vi "Viavi - Get Measure Data.vi"(8 "error in (no error)":errorcluster, 9 "Selected Wavelength":bool, 10 "Warning/Error Params":T3={"IL Param"={"Warning High"=inf, "Warning Low"=-inf, "Fail High"=inf, "Fail Low"=-inf, "Display Precision"=0}, "RL Param"={"Warning High"=inf, "Warning Low"=-inf, "Fail High"=inf, "Fail Low"=-inf, "Display Precision"=0}, "RL2 Param"={"Warning High"=inf, "Warning Low"=-inf, "Fail High"=inf, "Fail Low"=-inf, "Display Precision"=0}, "Power Param"={"Warning High"=inf, "Warning Low"=-inf, "Fail High"=inf, "Fail Low"=-inf, "Display Precision"=0}, "Length Param"={"Warning High"=inf, "Warning Low"=-inf, "Fail High"=inf, "Fail Low"=-inf, "Display Precision"=0}}, 11 "Viavi - strictRefs":T1) -> (0 "error out":errorcluster, 1 "Failure Output":string, 3 "Output Cluster":T2)   [LabVIEW 2017]
uses:
  Controls/Viavi - objectRefs.ctl
  <instrlib>/Viavi mORL-A1/Viavi mORL-A1.lvlib
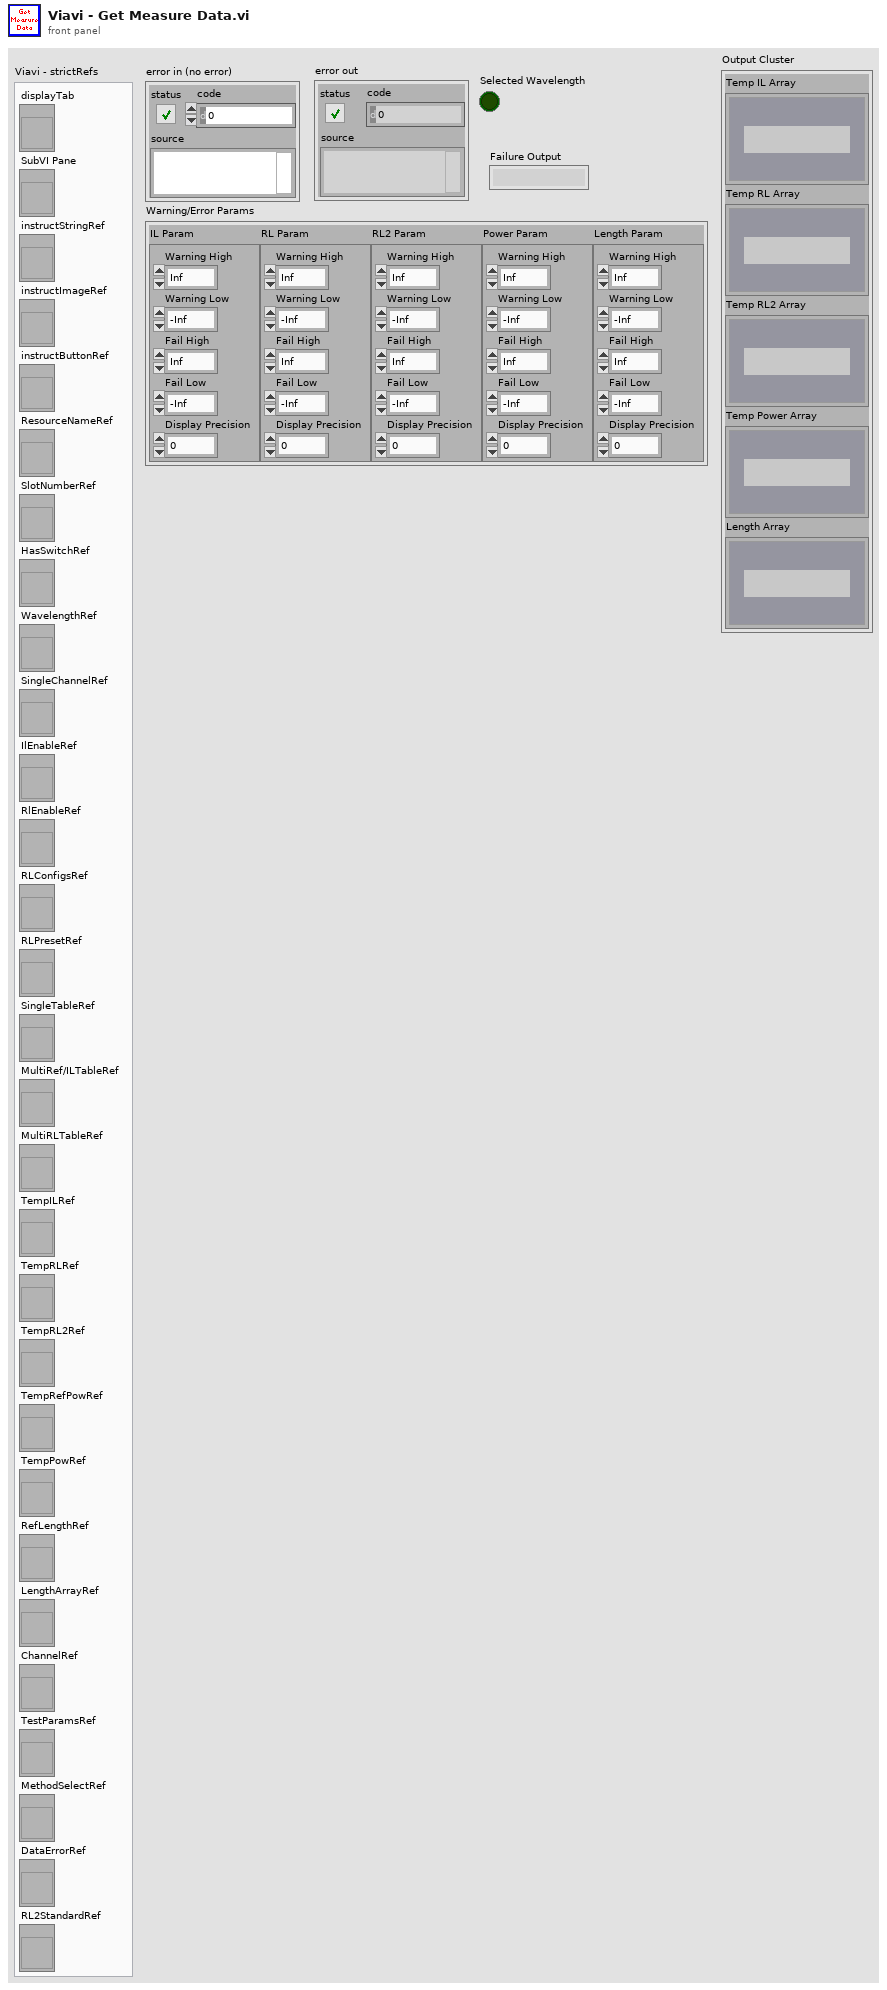
[diagram p1: front panel]
types:
  T1 = typedef "Viavi - objectRefs.ctl" = cluster{"displayTab":refnum<vi>, "SubVI Pane":refnum<vi>, "instructStringRef":refnum<vi>, "instructImageRef":refnum<vi>, "instructButtonRef":refnum<vi>, "ResourceNameRef":refnum<vi>, "SlotNumberRef":refnum<vi>, "HasSwitchRef":refnum<vi>, "WavelengthRef":refnum<vi>, "SingleChannelRef":refnum<vi>, "IlEnableRef":refnum<vi>, "RlEnableRef":refnum<vi>, "RLConfigsRef":refnum<vi>, "RLPresetRef":refnum<vi>, "SingleTableRef":refnum<vi>, "MultiRef/ILTableRef":refnum<vi>, "MultiRLTableRef":refnum<vi>, "TempILRef":refnum<vi>, "TempRLRef":refnum<vi>, "TempRL2Ref":refnum<vi>, "TempRefPowRef":refnum<vi>, "TempPowRef":refnum<vi>, "RefLengthRef":refnum<vi>, "LengthArrayRef":refnum<vi>, "ChannelRef":refnum<vi>, "TestParamsRef":refnum<vi>, "MethodSelectRef":refnum<vi>, "DataErrorRef":refnum<vi>, "RL2StandardRef":refnum<vi>}
  T2 = cluster{"Temp IL Array":cluster{"String":string, "Warning":bool, "Fail":bool, "Numeric":dbl}[], "Temp RL Array":cluster{"String":string, "Warning":bool, "Fail":bool, "Numeric":dbl}[], "Temp RL2 Array":cluster{"String":string, "Warning":bool, "Fail":bool, "Numeric":dbl}[], "Temp Power Array":cluster{"String":string, "Warning":bool, "Fail":bool, "Numeric":dbl}[], "Length Array":cluster{"String":string, "Warning":bool, "Fail":bool, "Numeric":dbl}[]}
  T3 = cluster{"IL Param":cluster{"Warning High":dbl, "Warning Low":dbl, "Fail High":dbl, "Fail Low":dbl, "Display Precision":i32}, "RL Param":cluster{"Warning High":dbl, "Warning Low":dbl, "Fail High":dbl, "Fail Low":dbl, "Display Precision":i32}, "RL2 Param":cluster{"Warning High":dbl, "Warning Low":dbl, "Fail High":dbl, "Fail Low":dbl, "Display Precision":i32}, "Power Param":cluster{"Warning High":dbl, "Warning Low":dbl, "Fail High":dbl, "Fail Low":dbl, "Display Precision":i32}, "Length Param":cluster{"Warning High":dbl, "Warning Low":dbl, "Fail High":dbl, "Fail Low":dbl, "Display Precision":i32}}
  T4 = enum32{"Left Anchor", "Right Anchor", "Center Anchor", "Left/Right Anchor", "Custom"}
  T5 = cluster{"String":string, "Warning":bool, "Fail":bool, "Numeric":dbl}[]
  T6 = cluster{"Measurement Mode":bool, "Enable RL2":bool, "RL1 Anchor Point":enum32{"Left DUT Connection", "Right DUT Connection", "Center on DUT"}, "RL1 Measure Points":cluster{"RL1 Left":dbl, "RL1 Right":dbl}, "RL2 Anchor Point":enum32{"Left DUT Connection", "Right DUT Connection", "Center on DUT"}, "RL2 Measure Points":cluster{"RL2 Left":dbl, "RL2 Right":dbl}}
  T7 = enum32{"Left DUT Connection", "Right DUT Connection", "Center on DUT"}
  T8 = cluster{"String":string, "Warning":bool, "Fail":bool, "Numeric":dbl}
  T9 = enum32{"Left/Right Anchor", "Left Anchor", "Right Anchor", "Center Anchor", "Custom"}
  T10 = cluster{"Warning High":dbl, "Warning Low":dbl, "Fail High":dbl, "Fail Low":dbl, "Display Precision":i32}
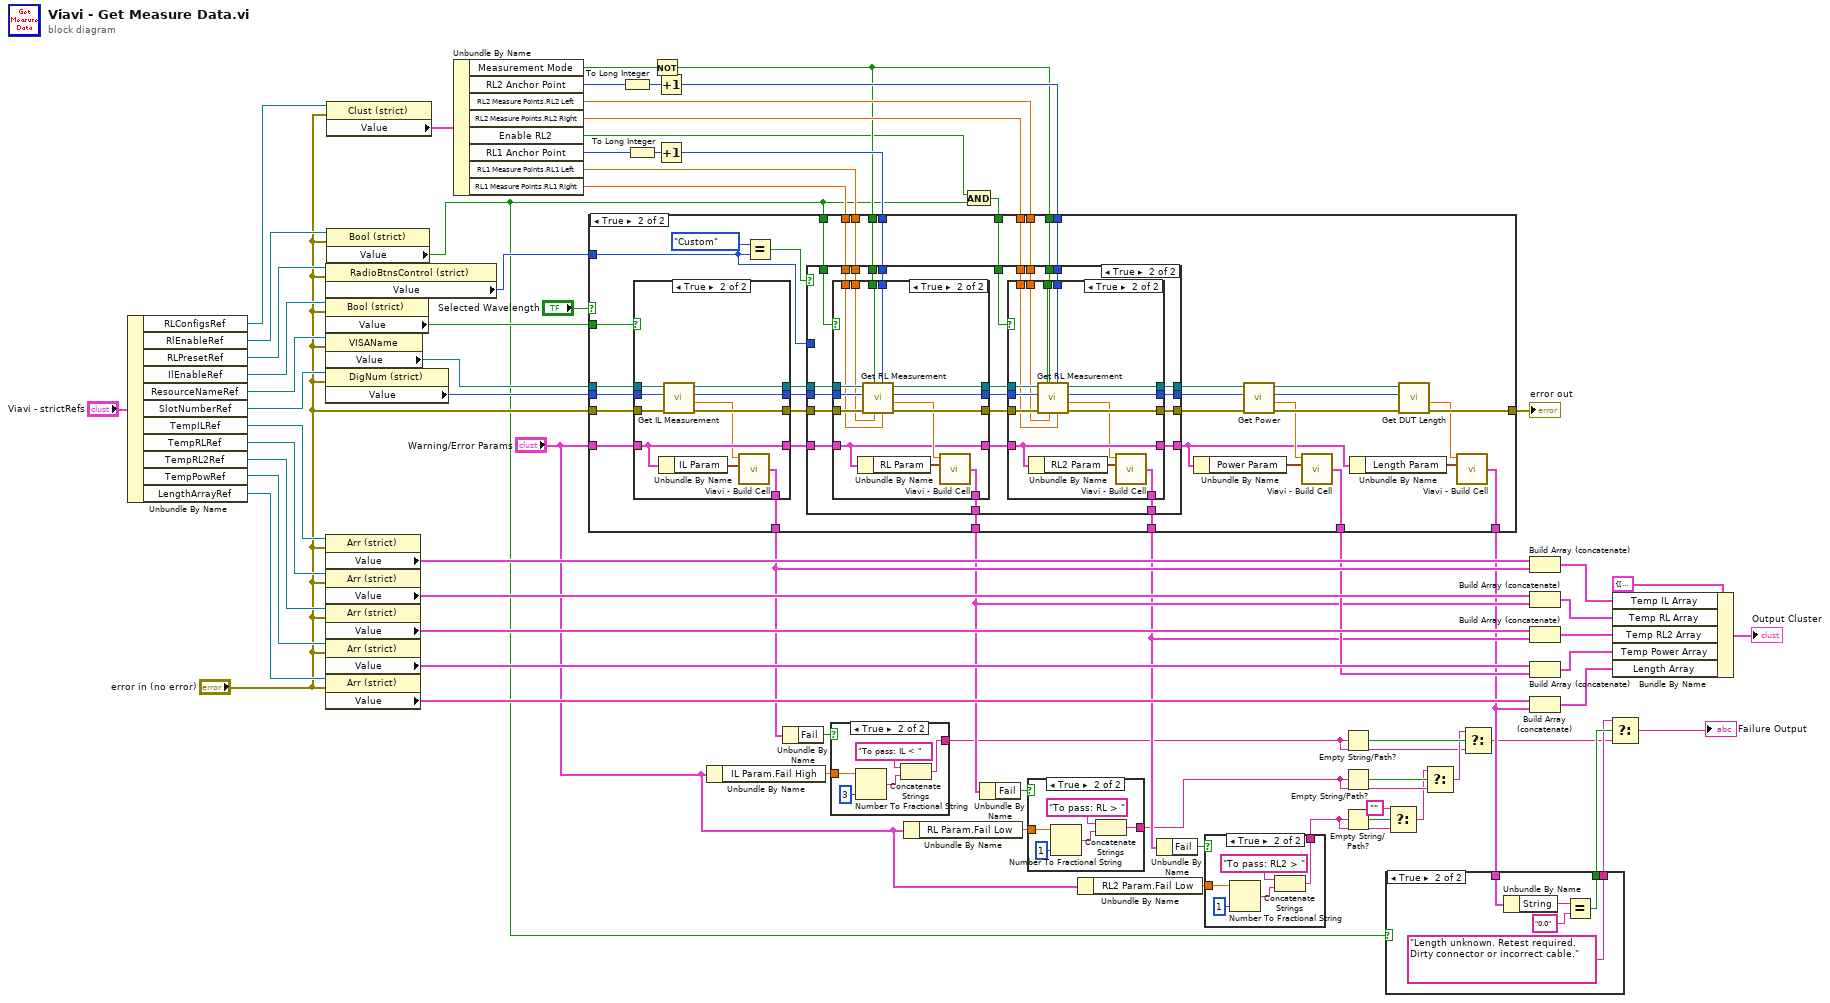
[diagram p0: block diagram]
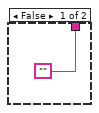
[diagram p3: hidden frame]
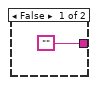
[diagram p4: hidden frame]
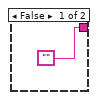
[diagram p5: hidden frame]
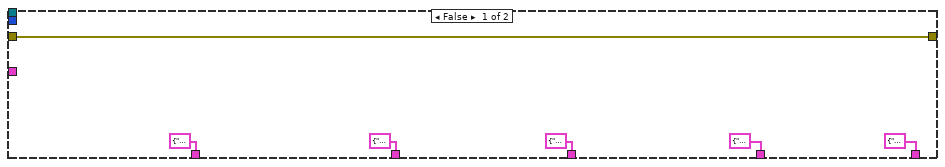
[diagram p6: hidden frame]
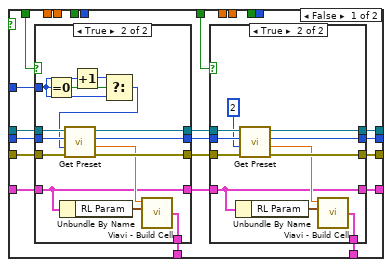
[diagram p7: hidden frame]
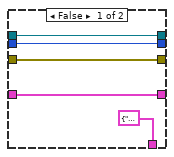
[diagram p8: hidden frame]
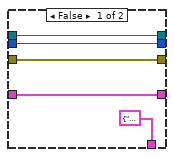
[diagram p9: hidden frame]
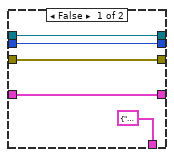
[diagram p10: hidden frame]
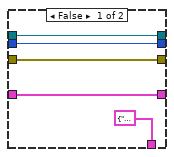
[diagram p11: hidden frame]
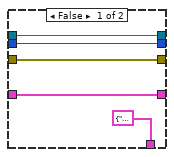
[diagram p12: hidden frame]
diagram:
  n1 = Unbundle By Name("Viavi - strictRefs") -> ("RLConfigsRef"=w29:refnum<vi>, "RlEnableRef"=w56:refnum<vi>, "RLPresetRef"=w45:refnum<vi>, "IlEnableRef"=w44:refnum<vi>, "ResourceNameRef"=w43:refnum<vi>, "SlotNumberRef"=w42:refnum<vi>, "TempILRef"=w41:refnum<vi>, "TempRLRef"=w40:refnum<vi>, "TempRL2Ref"=w39:refnum<vi>, "TempPowRef"=w38:refnum<vi>, "LengthArrayRef"=w37:refnum<vi>)
  n2 = property class="RadioBtnsControl (strict)"(reference=w45, error in="error in (no error)") -> ("Value"=w31:T4)  [unwired: 2 out]
  n3 = property class="Bool (strict)"(reference=w44, error in="error in (no error)") -> ("Value"=w2:bool)  [unwired: 2 out]
  n4 = property class="VISAName"(reference=w43, error in="error in (no error)") -> ("Value"=w71:refnum<visa-resource-name>)  [unwired: 2 out]
  n5 = property class="DigNum (strict)"(reference=w42, error in="error in (no error)") -> ("Value"=w72:i32)  [unwired: 2 out]
  n6 = property class="Arr (strict)"(reference=w41, error in="error in (no error)") -> ("Value"=w36:T5)  [unwired: 2 out]
  n7 = property class="Arr (strict)"(reference=w40, error in="error in (no error)") -> ("Value"=w35:T5)  [unwired: 2 out]
  n8 = property class="Arr (strict)"(reference=w39, error in="error in (no error)") -> ("Value"=w34:T5)  [unwired: 2 out]
  n9 = property class="Arr (strict)"(reference=w38, error in="error in (no error)") -> ("Value"=w33:T5)  [unwired: 2 out]
  n10 = property class="Arr (strict)"(reference=w37, error in="error in (no error)") -> ("Value"=w32:T5)  [unwired: 2 out]
  n11 = property class="Clust (strict)"(reference=w29, error in="error in (no error)") -> ("Value"=w30:T6)  [unwired: 2 out]
  n12 = property class="Bool (strict)"(reference=w56, error in="error in (no error)") -> ("Value"=w1:bool)  [unwired: 2 out]
  n13 = Unbundle By Name(w30) -> ("Measurement Mode"=w68:bool, "RL2 Anchor Point"=w65:T7, "RL2 Measure Points.RL2 Left"=w61:dbl, "RL2 Measure Points.RL2 Right"=w62:dbl, "Enable RL2"=w55:bool, "RL1 Anchor Point"=w67:T7, "RL1 Measure Points.RL1 Left"=w58:dbl, "RL1 Measure Points.RL1 Right"=w59:dbl)
  n14 = To Long Integer(number=w65) -> (32bit integer=w64:i32)
  n15 = To Long Integer(number=w67) -> (32bit integer=w66:i32)
  n16 = Not(x=w68) -> (.not. x?=w57:bool)
  n17 = Increment(x=w64) -> (x+1=w60:i32)
  n18 = Increment(x=w66) -> (x+1=w63:i32)
  n19 = Unbundle By Name("Warning/Error Params") -> ("IL Param.Fail High"=w24:dbl)
  n20 = Unbundle By Name("Warning/Error Params") -> ("RL Param.Fail Low"=w21:dbl)
  n21 = And(x=w55, y=w1) -> (x .and. y?=w54:bool)
  n22 = case shown="True" "Selected Wavelength" {
    tunnel: w72 -> [_ w114]
    tunnel: w71 -> [_ w113]
    tunnel: w2 -> [_ w106]
    tunnel: w1 -> [_ w105]
    tunnel: w54 -> [_ w104]
    tunnel: [w78 w103] -> w70
    tunnel: "error in (no error)" -> [w78 w102]
    tunnel: w59 -> [_ w101]
    tunnel: w58 -> [_ w100]
    tunnel: w63 -> [_ w99]
    tunnel: w62 -> [_ w98]
    tunnel: w61 -> [_ w97]
    tunnel: w60 -> [_ w96]
    tunnel: w57 -> [_ w95]
    tunnel: w57 -> [_ w94]
    tunnel: w31 -> [_ w92]
    tunnel: "Warning/Error Params" -> [_ w89]
    tunnel: [T8 {"String"="-.--", "Warning"=FALSE, "Fail"=FALSE, "Numeric"=0.0} ("Single Cell Cluster") w88] -> w27
    tunnel: [T8 {"String"="-.-", "Warning"=FALSE, "Fail"=FALSE, "Numeric"=0.0} ("Single Cell Cluster") w87] -> w22
    tunnel: [T8 {"String"="-.-", "Warning"=FALSE, "Fail"=FALSE, "Numeric"=0.0} ("Single Cell Cluster") w86] -> w17
    tunnel: [T8 {"String"="-.--", "Warning"=FALSE, "Fail"=FALSE, "Numeric"=0.0} ("Single Cell Cluster") w80] -> w26
    tunnel: [T8 {"String"="-.-", "Warning"=FALSE, "Fail"=FALSE, "Numeric"=0.0} ("Single Cell Cluster") w79] -> w7
    frame False {
    }
    frame True {
      n23 = case shown="True" w106 {
        tunnel: [w235 w245] -> w116
        tunnel: [w236 w246] -> w115
        tunnel: [w234 w244] -> w117
        tunnel: w114 -> [w235 w243]
        tunnel: w102 -> [w234 w242]
        tunnel: w113 -> [w236 w241]
        tunnel: [w233 w240] -> w90
        tunnel: w89 -> [w233 w240]
        tunnel: [T8 {"String"="-.--", "Warning"=FALSE, "Fail"=FALSE, "Numeric"=0.0} ("Single Cell Cluster") w237] -> w88
        frame False {
        }
        frame True {
          n24 = Unbundle By Name(w240) -> ("IL Param"=w238:T10)
          n25 = call <instrlib>:"Get IL Measurement.vi"("error in (no error)"=w242, "MAP-200 Slot Number"=w243, "VISA resource name"=w241) -> ("error out"=w244:errorcluster, "IL Return (db)"=w239:dbl, "MAP-200 Slot Number out"=w245:i32, "VISA resource name out"=w246:refnum<visa-resource-name>)  [unwired: 5 in]
          n26 = call "Viavi - Build Cell.vi"("Input Value"=w239, "Parameter Input"=w238) -> ("Single Cell Cluster"=w237:T8)  [unwired: 6 in]
        }
      }
      n27 = Equal?(x=T9."Custom", y=w92) -> (x = y?=w93:bool)
      n28 = case shown="True" w93 {
        tunnel: w117 -> [w127 w193]
        tunnel: w116 -> [w128 w192]
        tunnel: w115 -> [w129 w191]
        tunnel: [w124 w187] -> w112
        tunnel: [w125 w186] -> w111
        tunnel: [w126 w185] -> w110
        tunnel: w105 -> [w130 w184]
        tunnel: w104 -> [w131 w183]
        tunnel: w101 -> [_ w182]
        tunnel: w100 -> [_ w181]
        tunnel: w99 -> [_ w180]
        tunnel: w98 -> [_ w179]
        tunnel: w97 -> [_ w178]
        tunnel: w96 -> [_ w177]
        tunnel: w95 -> [_ w176]
        tunnel: w94 -> [_ w175]
        tunnel: w92 -> [w123 _]
        tunnel: [w120 w174] -> w81
        tunnel: w90 -> [w122 w172]
        tunnel: [w119 w171] -> w87
        tunnel: [w118 w170] -> w86
        frame False {
          n29 = case shown="True" w130 {
            tunnel: [w154 w164] -> w133
            tunnel: [w153 w166] -> w134
            tunnel: [w155 w165] -> w132
            tunnel: w128 -> [w154 w168]
            tunnel: w127 -> [w155 w169]
            tunnel: w129 -> [w153 w167]
            tunnel: w123 -> [_ w163]
            tunnel: [w152 w157] -> w121
            tunnel: w122 -> [w152 w157]
            tunnel: [T8 {"String"="-.-", "Warning"=FALSE, "Fail"=FALSE, "Numeric"=0.0} ("Single Cell Cluster") w156] -> w119
            frame False {
            }
            frame True {
              n30 = Equal To 0?(x=w163) -> (x = 0?=w161:bool)
              n31 = Unbundle By Name(w157) -> ("RL Param"=w159:T10)
              n32 = Increment(x=w163) -> (x+1=w162:T4)
              n33 = Select(t=w162, s=w161, f=w163) -> (s? t:f=w160:T4)
              n34 = call <instrlib>:"Get Preset.vi"("error in (no error)"=w169, "Preset Origin"=w160, "MAP-200 Slot Number"=w168, "VISA resource name"=w167) -> ("error out"=w165:errorcluster, "RL Return (dB)"=w158:dbl, "MAP-200 Slot Number out"=w164:i32, "VISA resource name out"=w166:refnum<visa-resource-name>)  [unwired: 4 in]
              n35 = call "Viavi - Build Cell.vi"("Input Value"=w158, "Parameter Input"=w159) -> ("Single Cell Cluster"=w156:T8)  [unwired: 6 in]
            }
          }
          n36 = case shown="True" w131 {
            tunnel: [w138 w148] -> w125
            tunnel: [w137 w149] -> w126
            tunnel: [w139 w147] -> w124
            tunnel: w133 -> [w138 w145]
            tunnel: w132 -> [w139 w146]
            tunnel: w134 -> [w137 w150]
            tunnel: w121 -> [w136 w141]
            tunnel: [w136 w141] -> w120
            tunnel: [T8 {"String"="-.-", "Warning"=FALSE, "Fail"=FALSE, "Numeric"=0.0} ("Single Cell Cluster") w140] -> w118
            frame False {
            }
            frame True {
              n37 = Unbundle By Name(w141) -> ("RL Param"=w143:T10)
              n38 = call <instrlib>:"Get Preset.vi"("error in (no error)"=w146, "Preset Origin"=2, "MAP-200 Slot Number"=w145, "VISA resource name"=w150) -> ("error out"=w147:errorcluster, "RL Return (dB)"=w142:dbl, "MAP-200 Slot Number out"=w148:i32, "VISA resource name out"=w149:refnum<visa-resource-name>)  [unwired: 4 in]
              n39 = call "Viavi - Build Cell.vi"("Input Value"=w142, "Parameter Input"=w143) -> ("Single Cell Cluster"=w140:T8)  [unwired: 6 in]
            }
          }
        }
        frame True {
          n40 = case shown="True" w184 {
            tunnel: [w216 w226] -> w189
            tunnel: [w215 w231] -> w190
            tunnel: [w217 w227] -> w188
            tunnel: w192 -> [w216 w229]
            tunnel: w193 -> [w217 w228]
            tunnel: w191 -> [w215 w230]
            tunnel: w181 -> [_ w222]
            tunnel: w182 -> [_ w225]
            tunnel: w176 -> [_ w224]
            tunnel: w180 -> [_ w223]
            tunnel: [w214 w220] -> w173
            tunnel: w172 -> [w214 w220]
            tunnel: [T8 {"String"="-.-", "Warning"=FALSE, "Fail"=FALSE, "Numeric"=0.0} ("Single Cell Cluster") w218] -> w171
            frame False {
            }
            frame True {
              n41 = Unbundle By Name(w220) -> ("RL Param"=w219:T10)
              n42 = call <instrlib>:"Get RL Measurement.vi"("Right Offset (m)"=w225, "Anchor Origins (See Block Diagram)"=w223, "Left Offset (m)"=w222, "Method (T = Discrete)"=w224, "error in (no error)"=w228, "MAP-200 Slot Number"=w229, "VISA resource name"=w230) -> ("error out"=w227:errorcluster, "RL Return (db)"=w221:dbl, "MAP-200 Slot Number out"=w226:i32, "VISA resource name out"=w231:refnum<visa-resource-name>)  [unwired: 1 in]
              n43 = call "Viavi - Build Cell.vi"("Input Value"=w221, "Parameter Input"=w219) -> ("Single Cell Cluster"=w218:T8)  [unwired: 6 in]
            }
          }
          n44 = case shown="True" w183 {
            tunnel: [w197 w207] -> w186
            tunnel: [w196 w212] -> w185
            tunnel: [w198 w208] -> w187
            tunnel: w189 -> [w197 w210]
            tunnel: w188 -> [w198 w209]
            tunnel: w190 -> [w196 w211]
            tunnel: w178 -> [_ w206]
            tunnel: w179 -> [_ w205]
            tunnel: w175 -> [_ w204]
            tunnel: w177 -> [_ w203]
            tunnel: [w195 w202] -> w174
            tunnel: w173 -> [w195 w202]
            tunnel: [T8 {"String"="-.-", "Warning"=FALSE, "Fail"=FALSE, "Numeric"=0.0} ("Single Cell Cluster") w199] -> w170
            frame False {
            }
            frame True {
              n45 = Unbundle By Name(w202) -> ("RL2 Param"=w201:T10)
              n46 = call <instrlib>:"Get RL Measurement.vi"("Right Offset (m)"=w205, "Anchor Origins (See Block Diagram)"=w203, "Left Offset (m)"=w206, "Method (T = Discrete)"=w204, "error in (no error)"=w209, "MAP-200 Slot Number"=w210, "VISA resource name"=w211) -> ("error out"=w208:errorcluster, "RL Return (db)"=w200:dbl, "MAP-200 Slot Number out"=w207:i32, "VISA resource name out"=w212:refnum<visa-resource-name>)  [unwired: 1 in]
              n47 = call "Viavi - Build Cell.vi"("Input Value"=w200, "Parameter Input"=w201) -> ("Single Cell Cluster"=w199:T8)  [unwired: 6 in]
            }
          }
        }
      }
      n48 = Unbundle By Name(w81) -> ("Power Param"=w85:T10)
      n49 = call <instrlib>:"Get Power.vi"("error in (no error)"=w112, "MAP-200 Slot Number"=w111, "VISA resource name"=w110) -> ("error out"=w107:errorcluster, "Power Return (dBm)"=w84:dbl, "MAP-200 Slot Number out"=w108:i32, "VISA resource name out"=w109:refnum<visa-resource-name>)  [unwired: 5 in]
      n50 = call "Viavi - Build Cell.vi"("Input Value"=w84, "Parameter Input"=w85) -> ("Single Cell Cluster"=w80:T8)  [unwired: 6 in]
      n51 = Unbundle By Name(w81) -> ("Length Param"=w82:T10)
      n52 = call <instrlib>:"Get DUT Length.vi"("error in (no error)"=w107, "MAP-200 Slot Number"=w108, "VISA resource name"=w109) -> ("error out"=w103:errorcluster, "Length Return (m)"=w83:dbl)  [unwired: 5 in, 2 out]
      n53 = call "Viavi - Build Cell.vi"("Input Value"=w83, "Parameter Input"=w82) -> ("Single Cell Cluster"=w79:T8)  [unwired: 6 in]
    }
  }
  "error out" <- w70
  n54 = Unbundle By Name(w27) -> ("Fail"=w25:bool)
  n55 = case shown="True" w25 {
    tunnel: w24 -> [_ w251]
    tunnel: ["" w249] -> w8
    frame False {
    }
    frame True {
      n56 = Number To Fractional String(number=w251, precision (6)=i16 3) -> (F-format string=w250:string)  [unwired: 2 in]
      n57 = Concatenate Strings("To pass: IL < " ("string"), w250) -> (w249:string)
    }
  }
  n58 = Unbundle By Name(w22) -> ("Fail"=w23:bool)
  n59 = case shown="True" w23 {
    tunnel: w21 -> [_ w257]
    tunnel: ["" w255] -> w11
    frame False {
    }
    frame True {
      n60 = Number To Fractional String(number=w257, precision (6)=i16 1) -> (F-format string=w256:string)  [unwired: 2 in]
      n61 = Concatenate Strings("To pass: RL > " ("string"), w256) -> (w255:string)
    }
  }
  n62 = Unbundle By Name("Warning/Error Params") -> ("RL2 Param.Fail Low"=w19:dbl)
  n63 = Unbundle By Name(w17) -> ("Fail"=w20:bool)
  n64 = case shown="True" w20 {
    tunnel: w19 -> [_ w263]
    tunnel: ["" w261] -> w13
    frame False {
    }
    frame True {
      n65 = Number To Fractional String(number=w263, precision (6)=i16 1) -> (F-format string=w262:string)  [unwired: 2 in]
      n66 = Concatenate Strings("To pass: RL2 > " ("string"), w262) -> (w261:string)
    }
  }
  n67 = Empty String/Path?(string/path=w8) -> (empty?=w16:bool)
  n68 = Empty String/Path?(string/path=w11) -> (empty?=w15:bool)
  n69 = Empty String/Path?(string/path=w13) -> (empty?=w14:bool)
  n70 = case shown="True" w1 {
    tunnel: w7 -> [_ w269]
    tunnel: [_ w266] -> w6
    tunnel: [_ "Length unknown. Retest required. Dirty connector or incorrect cable." ("string")] -> w5
    frame False {
    }
    frame True {
      n71 = Unbundle By Name(w269) -> ("String"=w267:string)
      n72 = Equal?(x=w267, y="0.0" ("string")) -> (x = y?=w266:bool)
    }
  }
  n73 = Select(t="", s=w14, f=w13) -> (s? t:f=w10:string)
  n74 = Select(t=w10, s=w15, f=w11) -> (s? t:f=w9:string)
  n75 = Select(t=w9, s=w16, f=w8) -> (s? t:f=w4:string)
  n76 = Build Array (concatenate)(w36, w27) -> (w47:T5)
  n77 = Build Array (concatenate)(w35, w22) -> (w48:T5)
  n78 = Build Array (concatenate)(w34, w17) -> (w49:T5)
  n79 = Build Array (concatenate)(w33, w26) -> (w50:T5)
  n80 = Build Array (concatenate)(w32, w7) -> (w51:T5)
  n81 = Select(t=w5, s=w6, f=w4) -> (s? t:f=→"Failure Output":string)
  n82 = Bundle By Name(cluster=T2 {"Temp IL Array"=[], "Temp RL Array"=[], "Temp RL2 Array"=[], "Temp Power Array"=[], "Length Array"=[]} ("Output Cluster"), "Temp IL Array"=w47, "Temp RL Array"=w48, "Temp RL2 Array"=w49, "Temp Power Array"=w50, "Length Array"=w51) -> (→"Output Cluster":T2)
